vi "Revolver Ocelot Main.vi"(8 "Ocelot":bool, 9 "Z":dbl(knob) scale=-1.0..1.0, 10 "Y":dbl(slide) scale=-1.0..1.0, 11 "X":dbl(slide) scale=-1.0..1.0) -> (0 "BRD":dbl(slide) scale=-1.0..1.0, 1 "BLD":dbl(slide) scale=-1.0..1.0, 2 "FRD":dbl(slide) scale=-1.0..1.0, 3 "FLD":dbl(slide) scale=-1.0..1.0, 4 "BRS":dbl(knob) scale=0.0..360.0, 5 "FRS":dbl(knob) scale=0.0..360.0, 6 "BLS":dbl(knob) scale=0.0..360.0, 7 "FLS":dbl(knob) scale=0.0..360.0)   [LabVIEW 2012]
panel:
  out "x/y":dbl
  in  "Max Velocity (in/sec)":dbl
  in  "Width of Chassis (in)":dbl
  in  "Length Of Chassis (in)":dbl
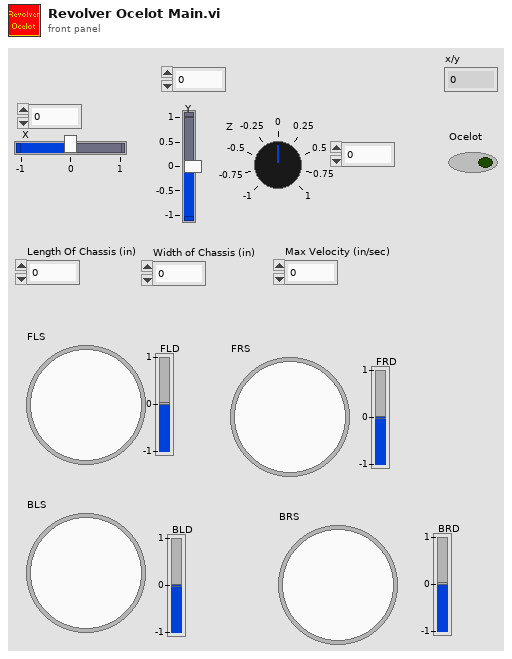
[diagram p1: front panel]
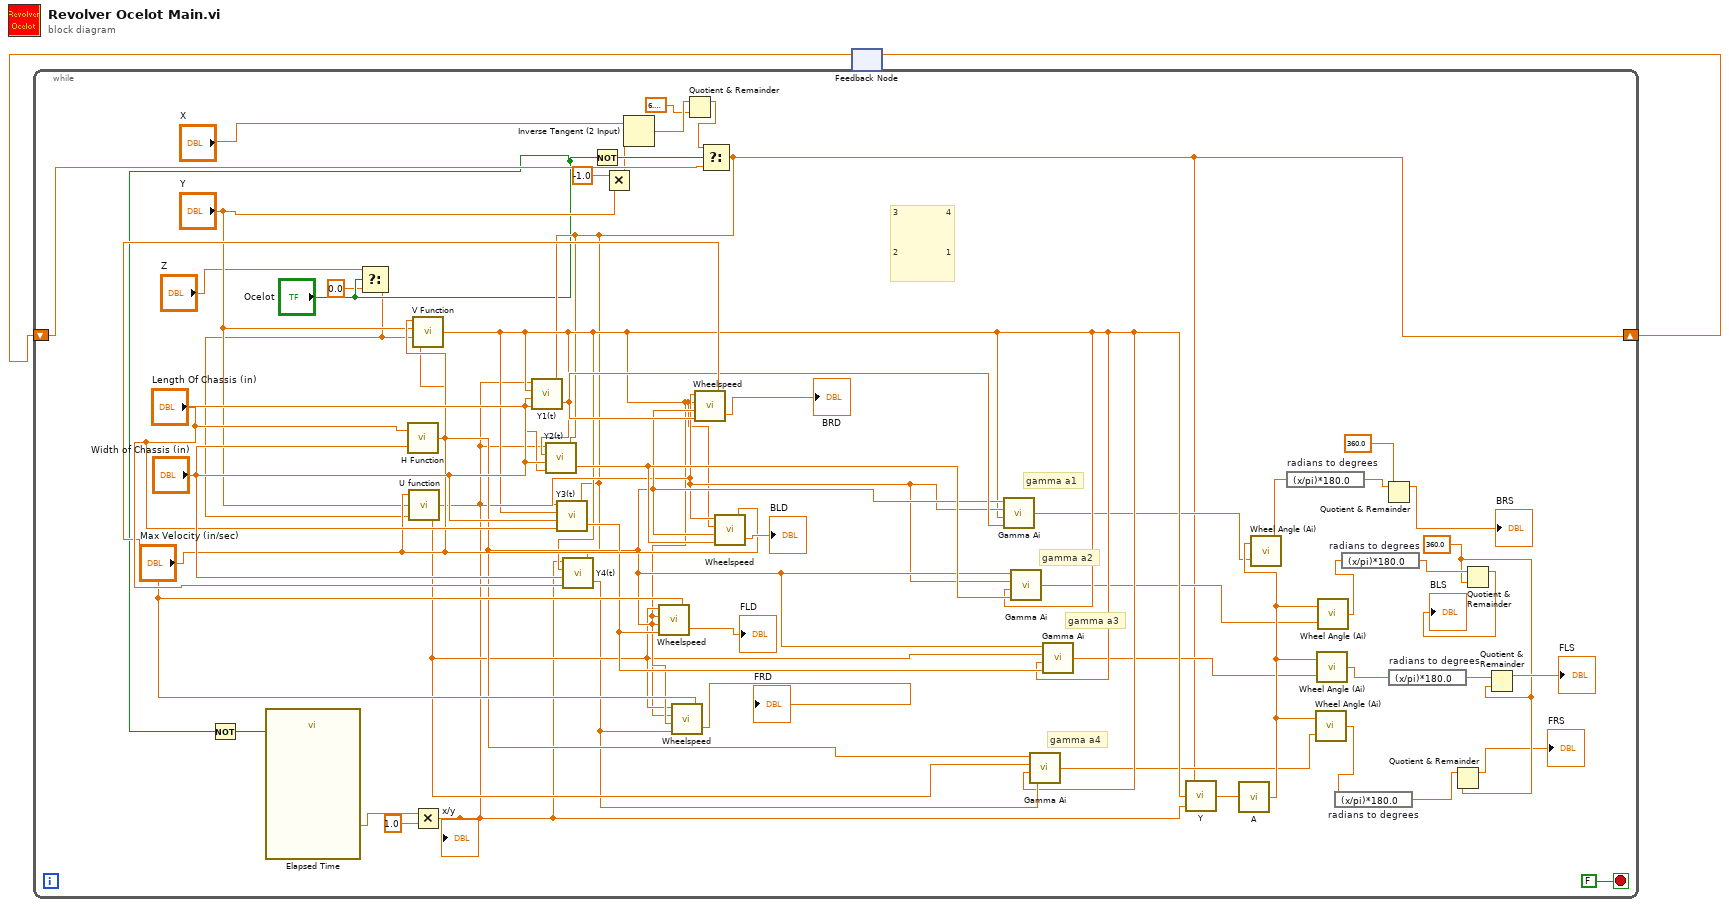
[diagram p0: block diagram]
diagram:
  n1 = feedback #1() -> (w1:dbl)  [unwired: 1 in]
  n2 = while {
    shift-right: [w29] -> w2
    shift-left: w1 -> [w32]
    stop <- FALSE stop-if-true
    w10 = 360.0 ("y")
    # "gamma a4"
    # "gamma a3"
    # "gamma a2"
    # "gamma a1"
    # "3                4\n\n\n\n2                1"
    n3 = Not(x="Ocelot") -> (.not. x?=w22:bool)
    n4 = call "Elapsed Time"("Reset"=w22) -> ("Elapsed Time (s)"=w31:dbl)  [unwired: 11 in, 7 out]
    n5 = Select(t="Z", s="Ocelot", f=0.0) -> (s? t:f=w4:dbl)
    n6 = call "H Function.vi"("Width"="Width of Chassis (in)", "Length"="Length Of Chassis (in)") -> ("h"=w45:dbl)
    n7 = call "U function.vi"("Z input"=w4, "Y input"="Y", "Max Velocity"="Max Velocity (in/sec)") -> ("U"=w44:dbl)
    n8 = call "V Function.vi"("H input"=w45, "Z input"=w4, "Y input"="Y", "Max Velocity"="Max Velocity (in/sec)") -> ("V"=w42:dbl)
    n9 = Multiply(x=w31, y=1.0) -> (x*y=w30:dbl)
    "x/y" <- w30
    n10 = Not(x="Ocelot") -> (.not. x?=w23:bool)
    n11 = Multiply(x=-1.0, y="Y") -> (x*y=w8:dbl)
    n12 = Inverse Tangent (2 Input)(1:w8, 2:"X") -> (0:w21:dbl)
    n13 = Quotient & Remainder(x=w21, y=6.283185307179586) -> (x-y*floor(x/y)=w19:dbl)  [unwired: 1 out]
    n14 = Select(t=w19, s=w23, f=w32) -> (s? t:f=w29:dbl)
    n15 = call "Y1(t).vi"("Initial Position"=w29, "L"="Length Of Chassis (in)", "W"="Width of Chassis (in)", "V"=w42, "T"=w30) -> ("Y1(t)"=w48:dbl)
    n16 = call "Y2(t).vi"("Initial Position"=w29, "L"="Length Of Chassis (in)", "W"="Width of Chassis (in)", "V"=w42, "T"=w30) -> ("Y2(t)"=w47:dbl)
    n17 = call "Y3(t).vi"("Initial Position"=w29, "L"="Length Of Chassis (in)", "W"="Width of Chassis (in)", "V"=w42, "T"=w30) -> ("Y3(t)"=w46:dbl)
    n18 = call "Y4(t).vi"("Initial Position"=w29, "L"="Length Of Chassis (in)", "W"="Width of Chassis (in)", "V"=w42, "T"=w30) -> ("Y4(t)"=w43:dbl)
    n19 = call "Wheelspeed.vi"("Max Speed"="Max Velocity (in/sec)", "Yi(t)"=w46, "H"=w45, "V"=w42, "U"=w44) -> ("Wheelspeed"=→"FLD":dbl)
    n20 = call "Wheelspeed.vi"("Max Speed"="Max Velocity (in/sec)", "Yi(t)"=w43, "H"=w45, "V"=w42, "U"=w44) -> ("Wheelspeed"=→"FRD":dbl)
    n21 = call "Wheelspeed.vi"("Max Speed"="Max Velocity (in/sec)", "Yi(t)"=w48, "H"=w45, "V"=w42, "U"=w44) -> ("Wheelspeed"=→"BRD":dbl)
    n22 = call "Wheelspeed.vi"("Max Speed"="Max Velocity (in/sec)", "Yi(t)"=w47, "H"=w45, "V"=w42, "U"=w44) -> ("Wheelspeed"=→"BLD":dbl)
    n23 = call "Gamma Ai.vi"("Yi(t)"=w48, "V"=w42, "U"=w44, "H"=w45) -> ("Gamma ai"=w39:dbl)
    n24 = call "Gamma Ai.vi"("Yi(t)"=w47, "V"=w42, "U"=w44, "H"=w45) -> ("Gamma ai"=w38:dbl)
    n25 = call "Gamma Ai.vi"("Yi(t)"=w43, "V"=w42, "U"=w44, "H"=w45) -> ("Gamma ai"=w36:dbl)
    n26 = call "Gamma Ai.vi"("Yi(t)"=w46, "V"=w42, "U"=w44, "H"=w45) -> ("Gamma ai"=w37:dbl)
    n27 = call "Y.vi"("T"=w30, "V"=w42, "Y(0)"=w29) -> ("Y"=w41:dbl)
    n28 = call "A.vi"("Y"=w41) -> ("A"=w40:dbl)
    n29 = call "Wheel Angle (Ai).vi"("Gamma ai"=w39, "A"=w40) -> ("Ai"=w28:dbl)
    n30 = expression code="(x/pi)*180.0" "radians to degrees"(w28) -> (w18:dbl)
    n31 = call "Wheel Angle (Ai).vi"("Gamma ai"=w36, "A"=w40) -> ("Ai"=w25:dbl)
    n32 = call "Wheel Angle (Ai).vi"("Gamma ai"=w37, "A"=w40) -> ("Ai"=w26:dbl)
    n33 = call "Wheel Angle (Ai).vi"("Gamma ai"=w38, "A"=w40) -> ("Ai"=w27:dbl)
    n34 = expression code="(x/pi)*180.0" "radians to degrees"(w25) -> (w11:dbl)
    n35 = expression code="(x/pi)*180.0" "radians to degrees"(w27) -> (w15:dbl)
    n36 = Quotient & Remainder(x=w18, y=360.0) -> (x-y*floor(x/y)=→"BRS":dbl)  [unwired: 1 out]
    n37 = expression code="(x/pi)*180.0" "radians to degrees"(w26) -> (w13:dbl)
    n38 = Quotient & Remainder(x=w11, y=w10) -> (x-y*floor(x/y)=→"FRS":dbl)  [unwired: 1 out]
    n39 = Quotient & Remainder(x=w15, y=w10) -> (x-y*floor(x/y)=→"BLS":dbl)  [unwired: 1 out]
    n40 = Quotient & Remainder(x=w13, y=w10) -> (x-y*floor(x/y)=→"FLS":dbl)  [unwired: 1 out]
  }
  n41 = feedback-in #1(w2) -> ()
